vi "Set DMA wrapper.vi"(6 "pDMAout":T1, 7 "bAckEna":i32, 8 "error in (no error)":errorcluster caption="错误输入（无错误）", 9 "pDMAin":T1, 10 "dwCanNodeId":u32, 11 "dwDevIndex":u32) -> (0 "error out":errorcluster caption="错误输出", 1 "pDMAin out":T1, 3 "function return":u32, 4 "pDMAout out":T1)   [LabVIEW 2016, in "UISimCanFunc_wrapper.lvlib"]
doc: "_declspec (dllexport) DWORD SetDMA_wrapper(DWORD dwDevIndex, DWORD dwCanNodeId, P_DMA_OBJ pDMAin, BOOL bAckEna, P_DMA_OBJ pDMAout);"
uses:
  <userlib>/UISimCanFunc_wrapper/UISimCanFunc_wrapper.lvlib
  <userlib>/UISimCanFunc_wrapper/UISimCanFunc_wrapper.dll
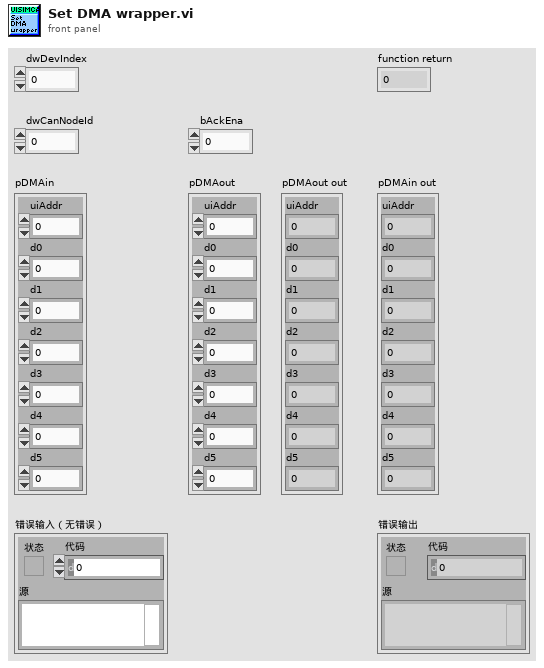
[diagram p1: front panel]
types:
  T1 = cluster{"uiAddr":u32, "d0":u8, "d1":u8, "d2":u8, "d3":u8, "d4":u8, "d5":u8}
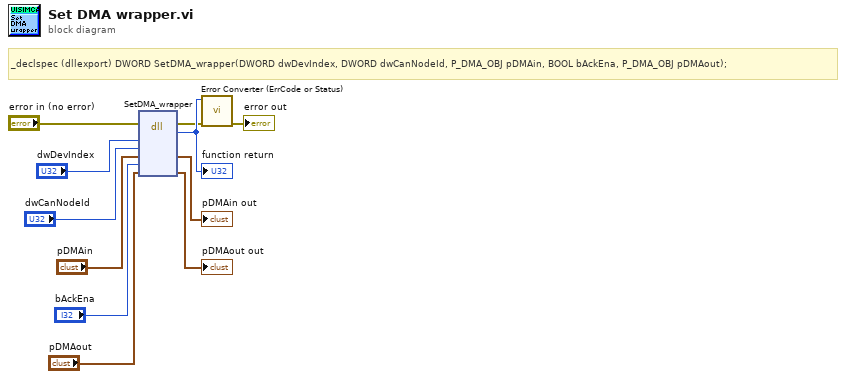
[diagram p0: block diagram]
diagram:
  # "_declspec (dllexport) DWORD SetDMA_wrapper(DWORD dwDevIndex, DWORD dwCanNodeId, P_DMA_OBJ pDMAin, BOOL bAckEna, P_DMA_OBJ pDMAout);"
  n1 = dll-call lib="C:/Program Files (x86)/National Instruments/LabVIEW 2016/user.lib/UISimCanFunc_wrapper/UISimCanFunc_wrapper.*" fn="SetDMA_wrapper"(error in="error in (no error)", "dwDevIndex"="dwDevIndex", "dwCanNodeId"="dwCanNodeId", "pDMAin"="pDMAin", "bAckEna"="bAckEna", "pDMAout"="pDMAout") -> (error out=w2:errorcluster, w11:u32, "pDMAin"=→"pDMAin out":T1, "pDMAout"=→"pDMAout out":T1)  [unwired: 5 in, 1 out]
  "function return" <- w11
  n2 = call <userlib>:"Error Converter (ErrCode or Status).vi"("error in (no error)"=w2, "error code"=w11) -> ("error out"=→"error out":errorcluster)  [unwired: 9 in]
